vi "Sensor Interface View.vi"(8 "error in (no error)":errorcluster, 11 "View Model":T1) -> (0 "error out":errorcluster, 3 "View Model":T1)   [LabVIEW 2017]
uses:
  View Model/Controls/View Model.ctl
  Configuration/Controls/Config Model.ctl
  Configuration/Controls/Config Data.ctl
  Error Handler/Controls/Error Model.ctl
  Error Handler/Controls/Error Data.ctl
  Error Handler/Controls/Error Type.ctl
  View Model/Controls/Shared Model.ctl
  Elevator Controller/Controls/Elevator Model.ctl
  Elevator Controller/Controls/Elevator Location.ctl
  Elevator Controller/Controls/Elevator CMD Data.ctl
  Elevator Controller/Controls/Elevator Commands.ctl
  Elevator Controller/Controls/Elevator Overhead.ctl
  Elevator Controller/Controls/Elevator States.ctl
panel:
  out "Elevator Position":i16(slide)=1 min=1 max=4 step=1 scale=1.0..4.0
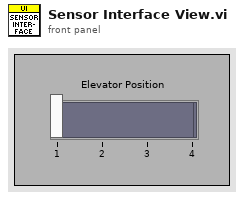
[diagram p1: front panel]
types:
  T1 = typedef "View Model.ctl" = cluster{"Config Model":T2, "Error Model":T3, "Shared Model":T4, "Elevator Model":T5}
  T2 = typedef "Config Model.ctl" = cluster{"Config Change":refnum<user-event>, "Config Data":refnum<data-value>}
  T3 = typedef "Error Model.ctl" = cluster{"Error Event":refnum<user-event>}
  T4 = typedef "Shared Model.ctl" = cluster{"Stop Event":refnum<user-event>, "Stop DVR":refnum<data-value>}
  T5 = typedef "Elevator Model.ctl" = cluster{"Motion Change":refnum<user-event>, "Direction Change":refnum<user-event>, "Door Position Change":refnum<user-event>, "Emergency Change":refnum<user-event>, "Floor Change":refnum<user-event>, "Elevator CMD":refnum<user-event>, "Controller Overhead":refnum<data-value>}
  T6 = typedef "Elevator Location.ctl" = enum16{"1st Floor", "2nd Floor", "3rd Floor", "4th Floor"}
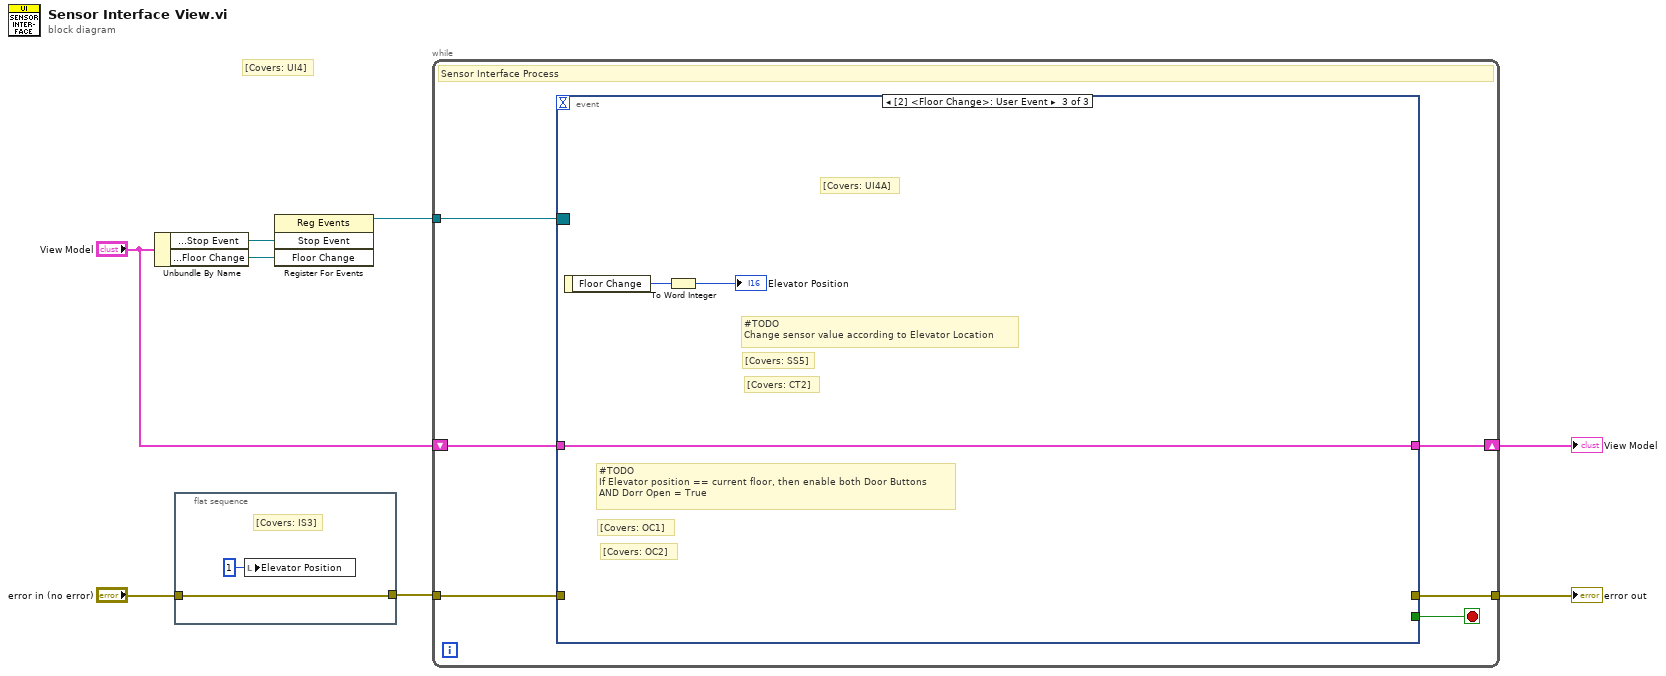
[diagram p0: block diagram]
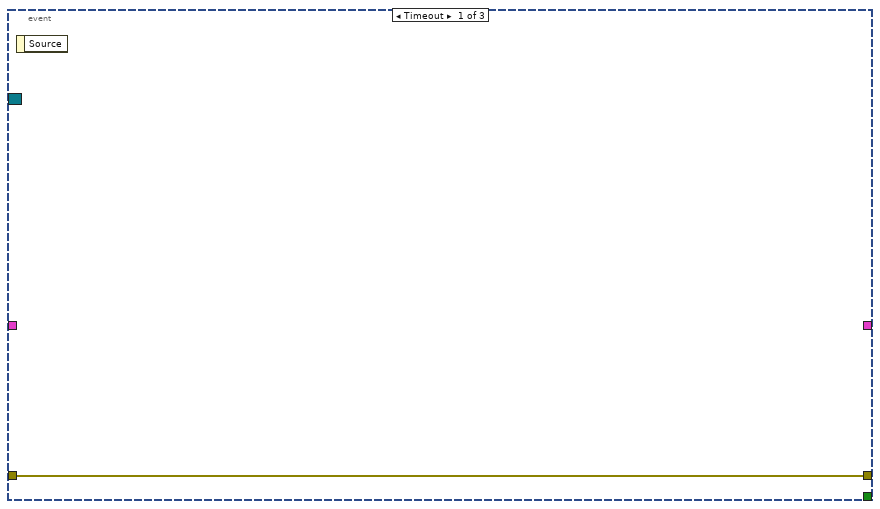
[diagram p2: hidden frame]
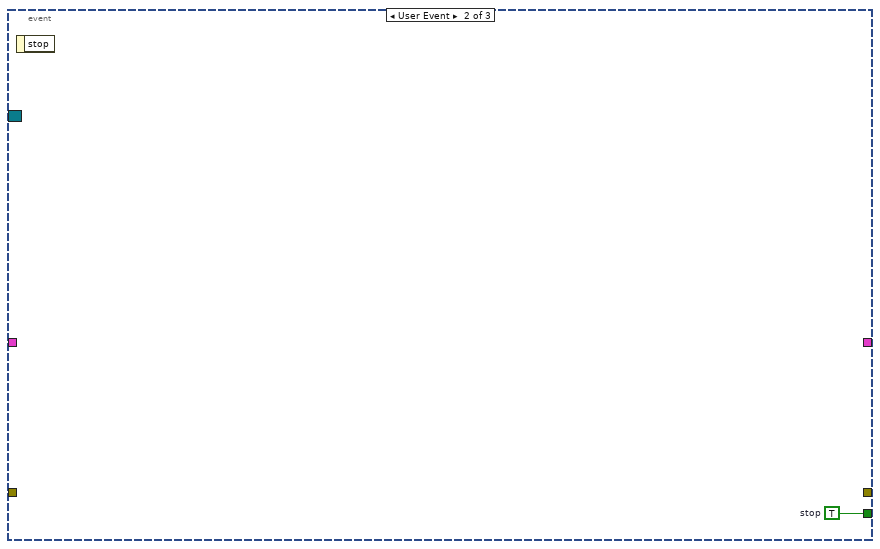
[diagram p3: hidden frame]
diagram:
  # "[Covers: UI4]"
  n1 = Unbundle By Name("View Model") -> ("Shared Model.Stop Event"=w8:refnum<user-event>, "Elevator Model.Floor Change"=w7:refnum<user-event>)
  n2 = flat-sequence {
    tunnel: "error in (no error)" -> [w10]
    tunnel: [w10] -> w1
    frame #0 {
      # "[Covers: IS3]"
      n3 = local write "Elevator Position"(i16 1 ("Elevator Position")) -> ()
    }
  }
  n4 = register-events(w8, w7) -> (reference out=w6:refnum<event-registration>)  [unwired: 2 in, 1 out]
  n5 = while {
    tunnel: w6 -> [w16]
    tunnel: w1 -> [w15]
    tunnel: [w14] -> w5
    shift-right: [w11] -> w3
    shift-left: "View Model" -> [w12]
    stop <- w13 stop-if-true
    # "Sensor Interface Process"
    n6 = event shown="[2] <Floor Change>: User Event" {
      selector: w16 -> [_ _ _]
      dyn-events: _ -> [_ _ _]
      timeout: _ -> [_ _ _]
      tunnel: w15 -> [w17 _ _]
      tunnel: [w17 _ _] -> w14
      tunnel: [_ w18 _] -> w13
      tunnel: w12 -> [_ _ w19]
      tunnel: [_ _ w19] -> w11
      event Timeout {
        n7 = event-data() -> ()  [unwired: 1 in, 1 out]
      }
      event User Event {
        w18 = TRUE  # stop
        n8 = event-data() -> ()  [unwired: 1 in, 1 out]
      }
      event User Event {
        # "[Covers: OC2]"
        # "[Covers: OC1]"
        # "#TODO\nIf Elevator position == current floor, then enable both Door Buttons\nAND Dorr Open = True"
        # "[Covers: CT2]"
        # "#TODO\nChange sensor value according to Elevator Location"
        # "[Covers: SS5]"
        # "[Covers: UI4A]"
        n9 = event-data() -> ("Floor Change"=w21:T6)  [unwired: 1 in]
        n10 = To Word Integer(number=w21) -> (16bit integer=→"Elevator Position":i16)
      }
    }
  }
  "error out" <- w5
  "View Model" <- w3
